vi "Int2Volt.vi"(8 "error in (no error)":errorcluster, 11 "AI Integer In":fxp<+/-,20,20>) -> (0 "error out":errorcluster, 3 "Voltage Out [V]":dbl)   [LabVIEW 2018, in "AI_read.lvlib"]
doc: "Convert integer Analog Input value into floating point voltage value.\nRefer to http://www.ni.com/pdf/manuals/376047c.pdf (Page-10) for more information."
uses:
  AI_read.lvlib
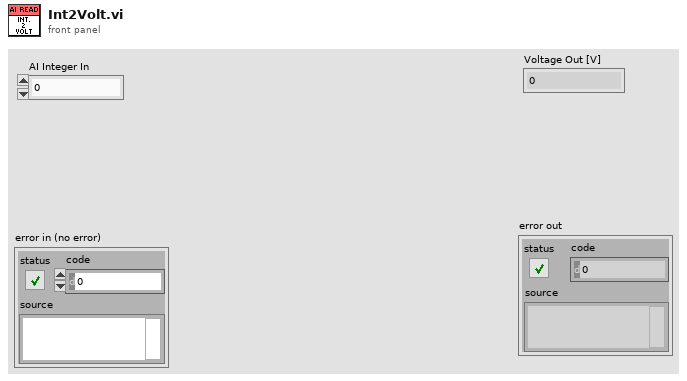
[diagram p1: front panel]
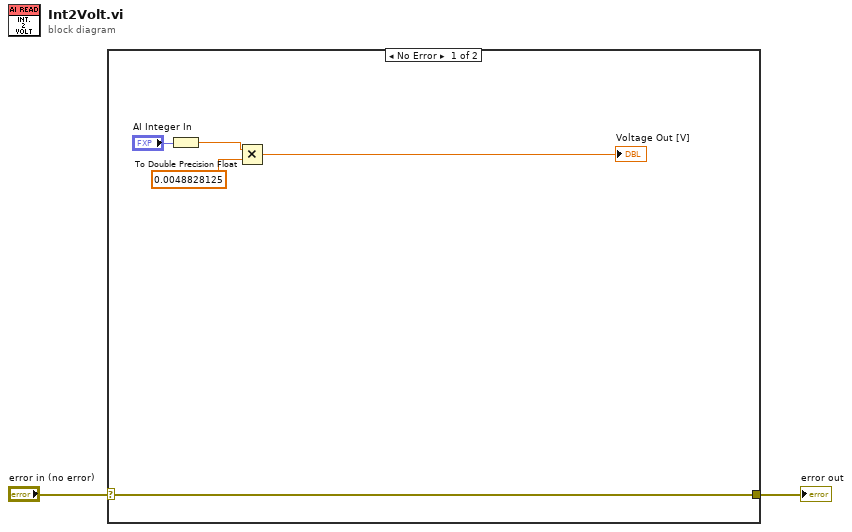
[diagram p0: block diagram]
diagram:
  n1 = case shown="No Error" "error in (no error)" {
    selector: "error in (no error)" -> [w7 w8]
    tunnel: [w7 w8] -> w1
    frame No Error {
      n2 = To Double Precision Float(number="AI Integer In") -> (double precision float=w5:dbl)
      n3 = Multiply(x=w5, y=0.0048828125) -> (x*y=→"Voltage Out [V]":dbl)
    }
    frame Error {
      # "Leave empty, this case is for error handling."
    }
  }
  "error out" <- w1
